vi "sub_Random U32.vi"(10 "lower bound":u32, 11 "upper bound":u32=100) -> (3 "number":u32)   [LabVIEW 2020]
doc: "Generates a random value from a specified range.\n\nThis VI returns a value greater than or equal to <b>lower bound</b> and less than <b>upper bound</b>. If <b>upper bound</b> is less than or equal to <b>lower bound</b>, this VI returns <b>lower bound</b>."
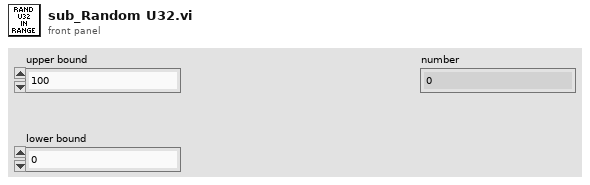
[diagram p1: front panel]
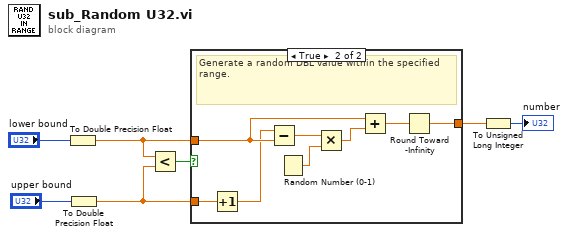
[diagram p0: block diagram]
diagram:
  n1 = To Double Precision Float(number="lower bound") -> (double precision float=w3:dbl)
  n2 = To Double Precision Float(number="upper bound") -> (double precision float=w2:dbl)
  n3 = Less?(x=w3, y=w2) -> (x < y?=w7:bool)
  n4 = case shown="True" w7 {
    tunnel: w3 -> [w8 w13]
    tunnel: w2 -> [_ w16]
    tunnel: [w8 w9] -> w4
    frame False {
      # "If bounds are reversed, always return the lower bound."
    }
    frame True {
      # "Generate a random DBL value within the specified range."
      n5 = Increment(x=w16) -> (x+1=w10:dbl)
      n6 = Subtract(x=w10, y=w13) -> (x-y=w15:dbl)
      n7 = Random Number (0-1)() -> (number: 0 to 1=w14:dbl)
      n8 = Multiply(x=w15, y=w14) -> (x*y=w12:dbl)
      n9 = Add(x=w13, y=w12) -> (x+y=w11:dbl)
      n10 = Round Toward -Infinity(1:w11) -> (0:w9:dbl)
    }
  }
  n11 = To Unsigned Long Integer(number=w4) -> (unsigned 32bit integer=→"number":u32)
